vi "Dark Correct.vi"(7 "Dark Array Model Path":path=path "C:/Users/dhstuart/Dropbox/CLTC/avantesSpectrometer/Cal Files/Dark Model Parameters.csv", 8 "error in (no error)":errorcluster, 9 "Counts":dbl[](array[numeric]), 11 "AVS Settings In":T1) -> (0 "error out":errorcluster, 1 "Counts normalize and dark corrected":dbl[](array[numeric]), 3 "AVS Settings Out":T1)   [LabVIEW 2014, in "AvaSpec.lvlib" / "Dark.lvlib"]
doc: "Read the dark model, parse out the model parameters, and apply the model to the raw data"
uses:
  Dark.lvlib
  Libraries/AS-5216-DLL/AVS settings.ctl
  <vilib>/Analysis/1siggen.llb/Ramp Pattern by Delta.vi
  <vilib>/Analysis/NI_AALBase.lvlib
  AvaSpec.lvlib
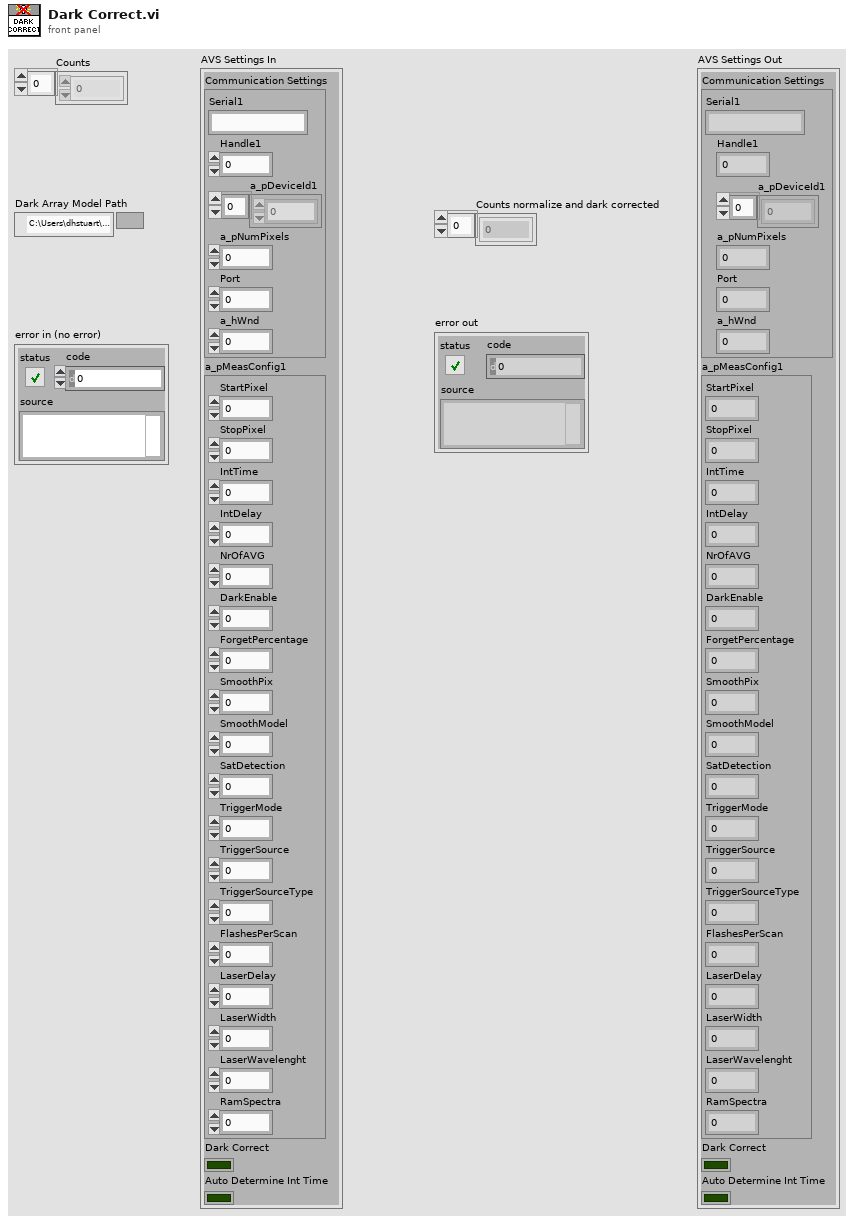
[diagram p1: front panel]
types:
  T1 = typedef "AvaSpec.lvlib/AVS settings.ctl" = cluster{"Communication Settings":cluster{"Serial1":string, "Handle1":i32, "a_pDeviceId1":u8[], "a_pNumPixels":u16, "Port":i32, "a_hWnd":i32}, "a_pMeasConfig1":cluster{"StartPixel":u16, "StopPixel":u16, "IntTime":sgl, "IntDelay":u32, "NrOfAVG":u32, "DarkEnable":u8, "ForgetPercentage":u8, "SmoothPix":u16, "SmoothModel":u8, "SatDetection":u8, "TriggerMode":u8, "TriggerSource":u8, "TriggerSourceType":u8, "FlashesPerScan":u16, "LaserDelay":u32, "LaserWidth":u32, "LaserWavelenght":sgl, "RamSpectra":u16}, "Dark Correct":bool, "Auto Determine Int Time":bool}
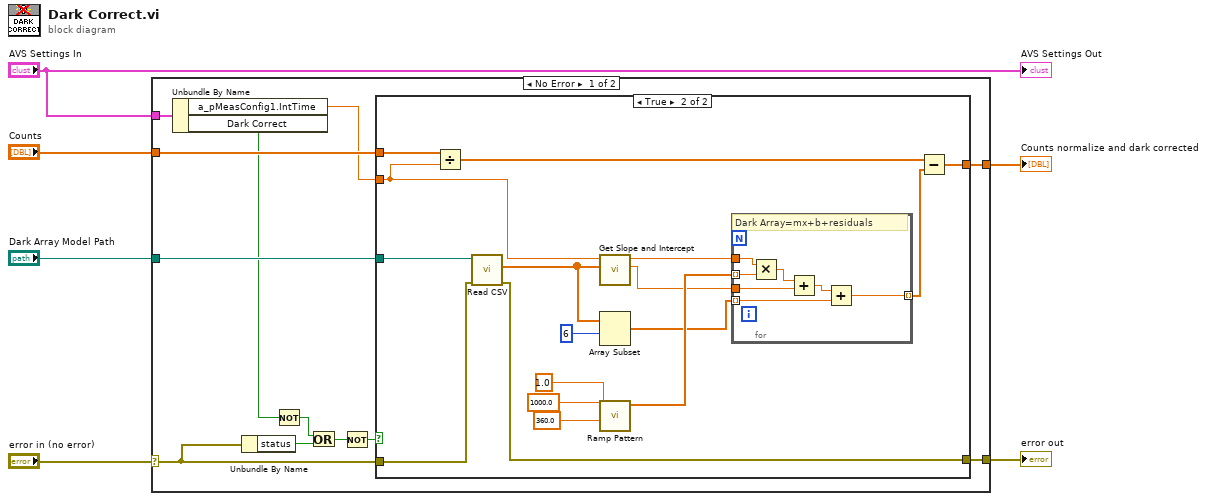
[diagram p0: block diagram]
diagram:
  n1 = case shown="No Error" "error in (no error)" {
    selector: "error in (no error)" -> [w7 w45]
    tunnel: "Dark Array Model Path" -> [w18 _]
    tunnel: "Counts" -> [w17 _]
    tunnel: [w16 _] -> w4
    tunnel: [w15 w45] -> w3
    tunnel: "AVS Settings In" -> [w13 _]
    frame No Error {
      n2 = Unbundle By Name(w13) -> ("a_pMeasConfig1.IntTime"=w14:sgl, "Dark Correct"=w11:bool)
      n3 = Unbundle By Name(w7) -> ("status"=w12:bool)
      n4 = Not(x=w11) -> (.not. x?=w10:bool)
      n5 = Or(x=w10, y=w12) -> (x .or. y?=w8:bool)
      n6 = Not(x=w8) -> (.not. x?=w9:bool)
      n7 = case shown="True" w9 {
        tunnel: w18 -> [_ w23]
        tunnel: w14 -> [_ w29]
        tunnel: w17 -> [w20 w30]
        tunnel: [w20 w26] -> w16
        tunnel: [w19 w21] -> w15
        tunnel: w7 -> [w19 w22]
        frame False {
        }
        frame True {
          n8 = Divide(x=w30, y=w29) -> (x/y=w28:dbl[])
          n9 = call "Read CSV.vi"("error in (no error)"=w22, "Path"=w23) -> ("error out"=w21:errorcluster, "first row"=w24:dbl[])  [unwired: 7 in, 1 out]
          n10 = call "Get Slope and Intercept.vi"("Read Dark File"=w24, "Integration Time"=w29) -> ("Intercept Out"=w31:dbl, "Slope Out"=w32:dbl)  [unwired: 8 in]
          n11 = Array Subset(array=w24, index=6) -> (w25:dbl[])  [unwired: 1 in]
          n12 = call-poly <vilib>:"Ramp Pattern.vi"("start"=360.0, "end"=1000.0, "delta"=1.0) -> ("Ramp Pattern"=w33:dbl[])  [unwired: 6 in, 2 out]
          n13 = for {
            tunnel: w25 -> [w39] mode=indexing
            tunnel: w33 -> [w43] mode=indexing
            tunnel: w32 -> [w44]
            tunnel: w31 -> [w41]
            tunnel: [w38] -> w27 mode=indexing
            # "Dark Array=mx+b+residuals"
            n14 = Multiply(x=w44, y=w43) -> (x*y=w42:dbl)
            n15 = Add(x=w42, y=w41) -> (x+y=w40:dbl)
            n16 = Add(x=w40, y=w39) -> (x+y=w38:dbl)
          }
          n17 = Subtract(x=w28, y=w27) -> (x-y=w26:dbl[])
        }
      }
    }
    frame Error {
    }
  }
  "error out" <- w3
  "Counts normalize and dark corrected" <- w4
  "AVS Settings Out" <- "AVS Settings In"
